vi "Remove SRs.vi"(8 "error in":errorcluster, 9 "entered SRs in":i32[](array[numeric]), 11 "Data Loop Data in":T1) -> (0 "error out":errorcluster, 3 "Data Loop Data out":T1)   [LabVIEW 2018]
uses:
  Type Defs/Data Loop Data.ctl
  Support/Message Queue/Message Cluster.ctl
  Support/Message Queue/Message Queue.lvlib
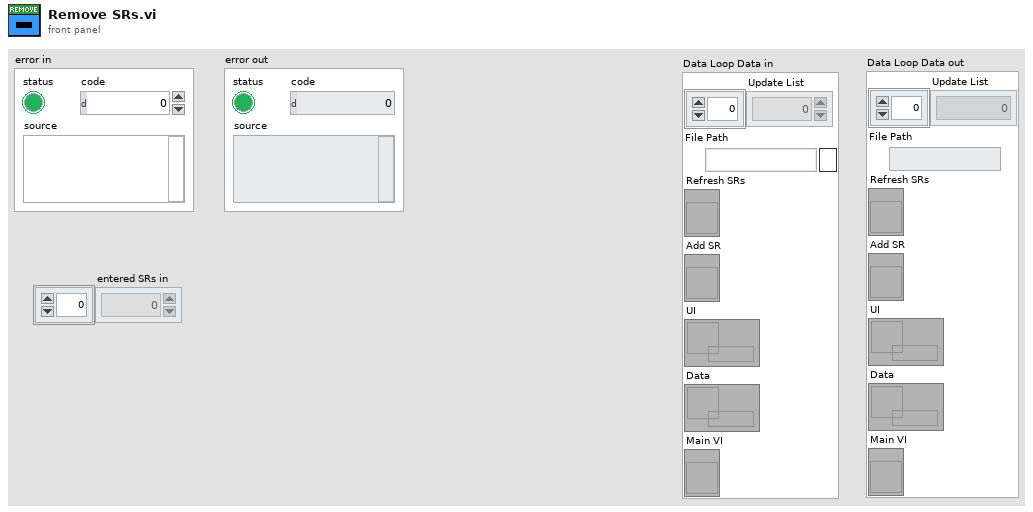
[diagram p1: front panel]
types:
  T1 = typedef "Data Loop Data.ctl" = cluster{"Update List":i32[], "File Path":path, "Refresh SRs":refnum<vi>, "Add SR":refnum<vi>, "UI":refnum<queue>, "Data":refnum<queue>, "Main VI":refnum<vi>}
  T2 = typedef "SR Cluster.ctl" = cluster{"Color":u32, "SR Number":i32, "SR Status":T3, "Name":string, "Summary":string, "Last Updated":timestamp, "SR Type":string, "Service Level":string, "Days Open":dbl, "Creation Date":timestamp}
  T3 = typedef "SR Status.ctl" = enum16{"Caller Abandoned", "Created in Error", "Expired", "Forum Resolved AE", "Forum Resolved Customer", "IN WORK", "IN WORK Collab with AES", "IN WORK Collab with PSE", "IN WORK Collab with SE", "IN WORK Customer Added Note", "IN WORK Escalation", "IN WORK Wait on Customer", "Open", "Potentially Resolved", "Presumed Resolved", "RMA Approved for Return", "RMA Closed", "RMA Closed - DOA", "RMA In Progress", "RMA Open", "RMA Waiting on Customer", "Resolved", "Passed Off"}
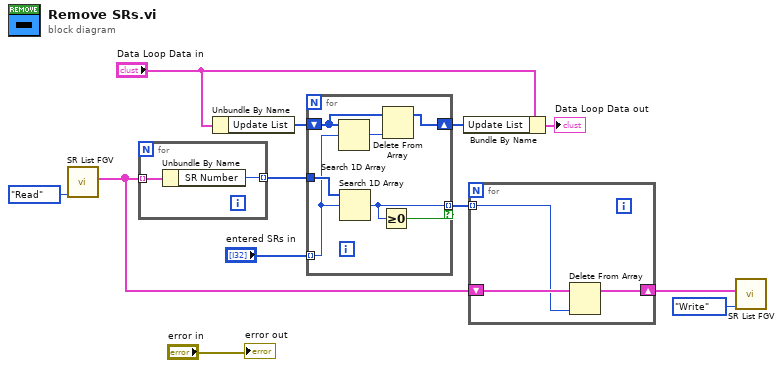
[diagram p0: block diagram]
diagram:
  n1 = call "SR List FGV.vi"("Operation"=enum16{"Initialize", "Write", "Read", "Clear"}."Read") -> ("list out"=w4:T2[])  [unwired: 9 in, 1 out]
  n2 = for {
    tunnel: w4 -> [w14] mode=indexing
    tunnel: [w13] -> w9 mode=indexing
    n3 = Unbundle By Name(w14) -> ("SR Number"=w13:i32)
  }
  n4 = Unbundle By Name("Data Loop Data in") -> ("Update List"=w7:i32[])
  n5 = for {
    tunnel: "entered SRs in" -> [w15] mode=indexing
    tunnel: w9 -> [w21]
    tunnel: [w20] -> w6 mode=indexing if=w19
    shift-right: [w16] -> w1
    shift-left: w7 -> [w18]
    n6 = Search 1D Array(1D array=w18, element=w15) -> (index of element=w17:i32)  [unwired: 1 in]
    n7 = Search 1D Array(1D array=w21, element=w15) -> (index of element=w20:i32)  [unwired: 1 in]
    n8 = Greater Or Equal To 0?(x=w20) -> (x >= 0?=w19:bool)
    n9 = Delete From Array(array=w18, index=w17) -> (array with subset deleted=w16:i32[])  [unwired: 1 in, 1 out]
  }
  n10 = Bundle By Name(cluster="Data Loop Data in", "Update List"=w1) -> (→"Data Loop Data out":T1)
  n11 = for {
    tunnel: w6 -> [w23] mode=indexing
    shift-right: [w22] -> w2
    shift-left: w4 -> [w24]
    n12 = Delete From Array(array=w24, index=w23) -> (array with subset deleted=w22:T2[])  [unwired: 1 in, 1 out]
  }
  n13 = call "SR List FGV.vi"("Operation"=enum16{"Initialize", "Write", "Read", "Clear"}."Write", "list in"=w2) -> ()  [unwired: 8 in, 2 out]
  "error out" <- "error in"
